vi "Receive Message.vi"(6 "priority":i32, 10 "Data Tracker in":refnum<class "Data Tracker.lvclass">, 11 "Message in":refnum<class "Message.lvclass">) -> (0 "error out":errorcluster, 2 "Actor out":refnum<class "Actor.lvclass">)   [LabVIEW 2020, in "Data Tracker.lvlib" / "Data Tracker.lvclass"]
doc: "Filters for Data messages and send/store these on named notifiers (named by Data alias). All other messages are handled normally.\n\nThis implementation filters for Data messages and stores the contained Data on the subscribing Tracker elements."
uses:
  Data Tracker.lvclass
  PPL/HDH.Actor Framework.Core.Actor.lvlibp/1abvi3w/vi.lib/ActorFramework/Message/Message.lvclass
  PPL/HDH.Actor Framework.Core.Actor.lvlibp/1abvi3w/vi.lib/ActorFramework/Actor/Actor.lvclass
  C:/Current projects/WS/PPL/HDH.Actor Framework.Core.Actor.lvlibp/1abvi3w/vi.lib/ActorFramework/Actor/Actor.lvclass
  PPL/HDH.Actor Framework.Core.Publisher.lvlibp/Messages/Data Msg/Data Msg.lvclass
  Data Tracker.lvclass/Data Tracker.ctl
  PPL/HDH.Data.Generic.lvlibp/Data.lvclass
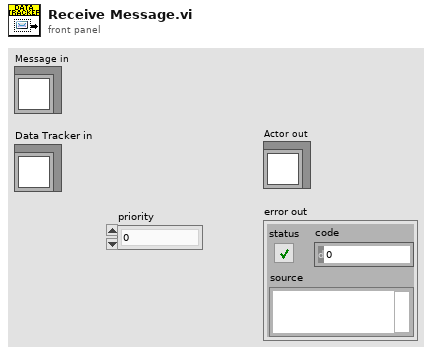
[diagram p1: front panel]
types:
  T1 = typedef "Data Tracker.lvlib/Data Tracker.lvclass/Ctl_Tracker Element.ctl" = cluster{"Tracker Type":refnum<class "Data Tracker Msg.lvclass">, "Subscriptions":refnum<class "Data.lvclass">[], "Data":refnum<class "Data.lvclass">[], "Size":u32, "Start Time":timestamp}
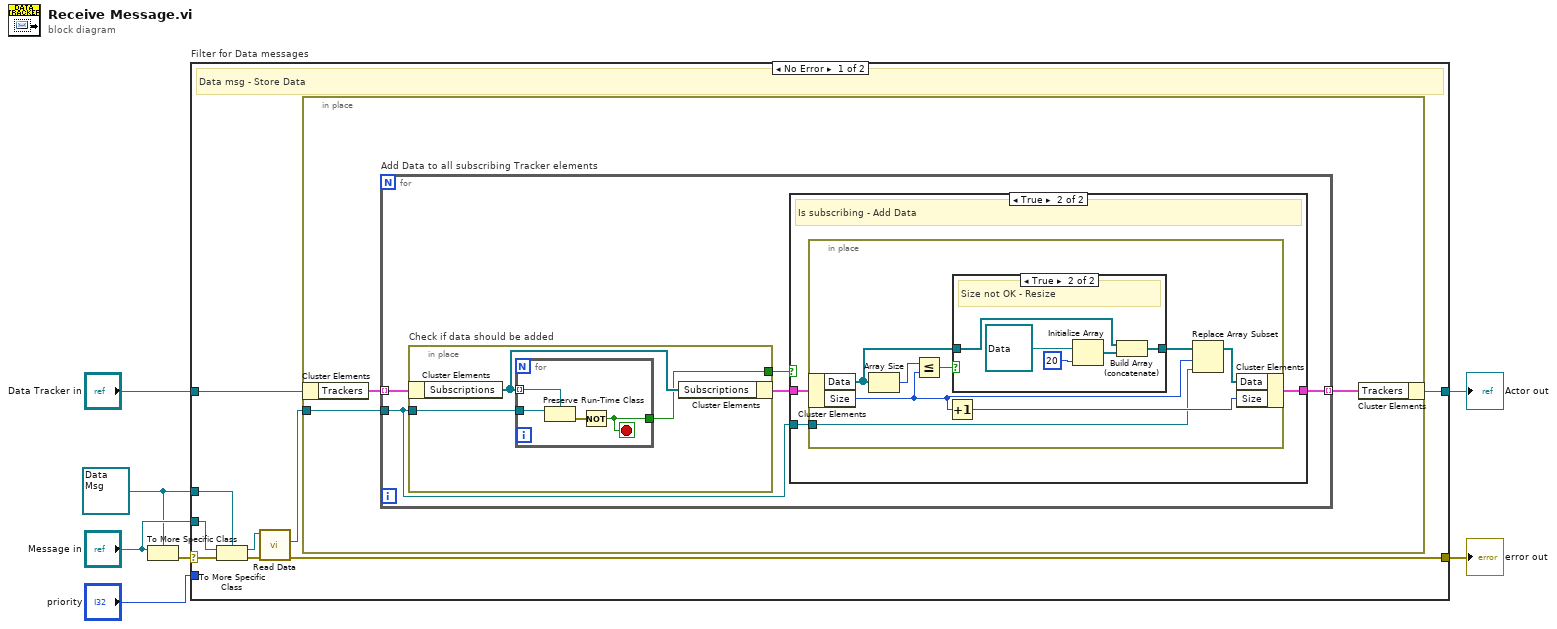
[diagram p0: block diagram]
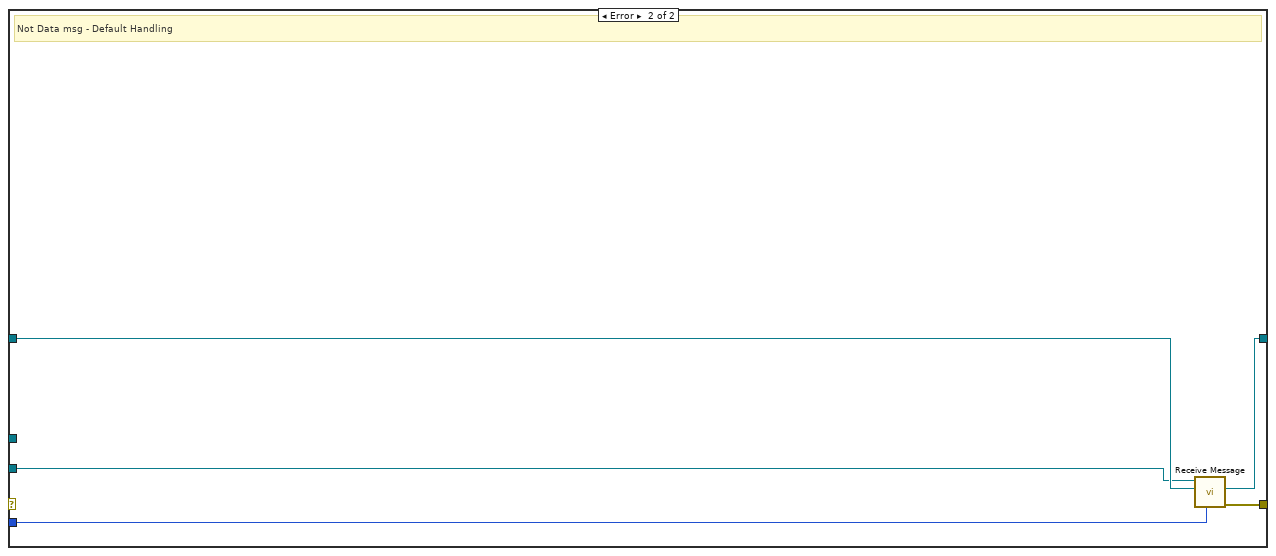
[diagram p4: hidden frame]
diagram:
  w1 = refnum<class "Data Msg.lvclass"> refnum ("HDH.Actor Framework.Core.Publisher.lvlibp:Data Msg.lvclass")
  n1 = To More Specific Class(target class=w1, reference="Message in") -> (error out=w3:errorcluster)  [unwired: 1 in, 1 out]
  n2 = case "Filter for Data messages" shown="No Error" w3 {
    selector: w3 -> [w14 _]
    tunnel: [w11 w54] -> w7
    tunnel: [w9 w53] -> w6
    tunnel: "priority" -> [_ w52]
    tunnel: "Data Tracker in" -> [w10 w51]
    tunnel: "Message in" -> [w16 w50]
    tunnel: w1 -> [w15 _]
    frame No Error {
      # "Data msg - Store Data"
      n3 = To More Specific Class(target class=w15, reference=w16, error in=w14) -> (specific class reference=w13:refnum<class "Data Msg.lvclass">, error out=w12:errorcluster)
      n4 = call "Read Data.vi"("error in (no error)"=w12, "Data Msg in"=w13) -> ("error out"=w11:errorcluster, "Data"=w8:refnum<class "Data.lvclass">)  [unwired: 7 in, 1 out]
      n5 = in-place {
        in-place-border: w8 -> [w18]
        n6 = in-place-cluster #1(w10) -> ("Trackers"=w19:T1[])
        n7 = for "Add Data to all subscribing Tracker elements" {
          tunnel: w19 -> [w24] mode=indexing
          tunnel: w18 -> [w22]
          tunnel: [w21] -> w17 mode=indexing
          n8 = in-place "Check if data should be added" {
            in-place-border: w22 -> [w45]
            in-place-border: [w43] -> w20
            n9 = in-place-cluster #2(w24) -> ("Subscriptions"=w44:refnum<class "Data.lvclass">[])
            n10 = for {
              tunnel: w45 -> [w49]
              tunnel: w44 -> [w48] mode=indexing
              tunnel: [w46] -> w43
              stop <- w46 stop-if-true
              n11 = Preserve Run-Time Class(object in=w49, 2:w48) -> (error out=w47:errorcluster)  [unwired: 1 in, 1 out]
              n12 = Not(x=w47) -> (.not. x?=w46:bool)
            }
            n13 = in-place-cluster #2("Subscriptions"=w44) -> (w23:T1)
          }
          n14 = case shown="True" w20 {
            tunnel: w23 -> [w25 w28]
            tunnel: w22 -> [_ w27]
            tunnel: [w25 w26] -> w21
            frame False {
              # "Is not subscribing - Do not add Data"
            }
            frame True {
              # "Is subscribing - Add Data"
              n15 = in-place {
                in-place-border: w27 -> [w32]
                n16 = in-place-cluster #3(w28) -> ("Data"=w33:refnum<class "Data.lvclass">[], "Size"=w29:u32)
                n17 = Array Size(array=w33) -> (size(s)=w30:i32)
                n18 = Less Or Equal?(x=w30, y=w29) -> (x <= y?=w36:bool)
                n19 = Increment(x=w29) -> (x+1=w35:u32)
                n20 = case shown="True" w36 {
                  tunnel: [w37 w38] -> w34
                  tunnel: w33 -> [w37 w40]
                  frame False {
                    # "Size OK - Do nothing"
                  }
                  frame True {
                    # "Size not OK - Resize"
                    n21 = Initialize Array(refnum<class "Data.lvclass"> refnum ("HDH.Data.Generic.lvlibp:Data.lvclass"), 20 ("dimension size")) -> (w39:refnum<class "Data.lvclass">[])
                    n22 = Build Array (concatenate)(w40, w39) -> (w38:refnum<class "Data.lvclass">[])
                  }
                }
                n23 = Replace Array Subset(array=w34, new element=w32, index=w29) -> (w31:refnum<class "Data.lvclass">[])
                n24 = in-place-cluster #3("Data"=w31, "Size"=w35) -> (w26:T1)
              }
            }
          }
        }
        n25 = in-place-cluster #1("Trackers"=w17) -> (w9:refnum<class "Data Tracker.lvclass">)
      }
    }
    frame Error {
      # "Not Data msg - Default Handling"
      n26 = call-parent "Receive Message.vi"("priority"=w52, "Actor in"=w51, "Message in"=w50) -> ("error out"=w54:errorcluster, "Actor out"=w53:refnum<class "Actor.lvclass">)  [unwired: 7 in]
    }
  }
  "error out" <- w7
  "Actor out" <- w6
